vi "T90 konfig.vi"() -> ()   [LabVIEW 2020, in "T90.lvlib"]
uses:
  T90.lvlib
  Visualisierungs Elemente/Auswahlfeld.ctl
  Visualisierungs Elemente/Zahlen-Eingabefeld.ctl
  Zustand Auswahl.ctl
  Visualisierungs Elemente/String - Eingabefeld.ctl
  Visualisierungs Elemente/Pfad-Eingabefeld.ctl
  Seiten/System Einstellungen V2/Konfig Gasflasche.ctl
  Seiten/System Einstellungen V2/Gasflasche Auswahl.ctl
  Seiten/FT-IR/FGV FT-IR Gasliste Aktionen.ctl
  Seiten/System Einstellungen V2/Aktion FGV Gasbottledefinition.ctl
  Aktion FGV T90.ctl
  T90 main.vi
  Seiten/FT-IR/FT-IR.lvlib
  Allgemein/allgemeine Sub-VIs.lvlib
  Sprachverwaltung/Sprachverwaltung.lvlib
  Seiten/System Einstellungen V2/System Einstellungen V2.lvlib
  Linearisierung V2/Gasteiler/Gasteiler.lvlib
panel:
  out "Einheit":string="-22Y3" caption="-21Y8"
  in  "Sollwert:":T1 format="%#_5g"
  in  "Bearbeiter:":T2
  in  "Stabilisierungszeit:":T1 format="%#_5g"
  in  "Gasflasche":T3 items=["----"=10000, "IAG O2"=0, "IAG C2H2"=1, "IAG C2H4"=2, "IAG NH3 200"=3, "IAG NH3 2000"=4, "IAG NH3 3000"=5, "IAG CO 5%"=6, "IAG Propane 2%"=7, "IAG NO 1000"=8, "IAG MG"=9, "IAG SO2"=10, "IAG C3H6"=11, "IAG CO2"=12, "IAG CO"=13, "IAG N2O"=14, "IAG N2O 100"=15, "IAG NO2 1000"=16, "IAG NO2 100"=17, "IAG CH4"=18, "IAG Propane"=19, "IAG NO 5000"=20, "Hansi"=21]
  in  "Konfig Gasflasche":T4 caption="Konfigurierte Gasflasche verwenden"
  in  "max. Responsetime:":T1 format="%#_5g"
  in  "Pfad":T5
  in  "Textname:":T2
  in  "Abschaltzeit:":T1 format="%#_5g"
  in  "Abweichung:":T1 format="%#_5g"
  in  "Abbrechen":bool
  in  "Start":bool
  in  "Modus:":T6=1 items=["Cal Gas", "Entnahmestelle"]
  in  "Gaskomponente:":T7 caption="Komponente:" items=["NO (350,3000) LP 191C", "NO2 (150) LP 191C (1of2)", "NO2 (2000) LP 191C (2of2)", "N2O (300) LP 191C (1of2)", "NH3 (300) LP 191C (1of2)", "NH3 (900,3000) LP 191C (2of2)", "HNCO (400) 191C", "H2O% (30) LP 191C", "Formaldehyde (70,500) LP 191C", "CO2 low% (4) LP 191C (2of2)", "CO2% (20) LP 191C (1of2)", "CO (700) LP 191C (1of3)", "CO% (1) LP 191C (2of3)", "Propylene (1000) LP 191C", "Aromatic HC C7 (500) LP 191C", "Ethylene (1000) LP 191C", "CH4 (250) LP 191C (1of2)", "CH4 (5000) LP 191C (2of2)", "Ethane (1000) LP 191C", "Acetylene (1000) LP 191C", "HNO2 (20) 191C", "MeOH (1000) 191C", "CO% (10) LP 191C (3of3)", "Formic Acid (100) 191C", "SO2 (500) LP 191C", "Acetaldehyde (1000) LP 191C", "COS (100) LP 191C", "1,3 butadiene (100) LP 191C", "Oil as Octane (200) LP 191C", "N2O (1000) LP 191C (2of2)", "Propane (200) LP 191C", "NO2 autorange (2000)", "CO autorange (100000)", "CH4 autorange (5000)", "NH3 autorange (3000)", "NOx autorange (3000)", "HCD (10000)", "NMHCD (10000)", "CO2% autorange (20)", "H2Oppm (300000)", "N2O autorange (1000)", "NMNEHCD (3000)", "Temp. Messzelle", "Druck Messzelle", "sBeam@2500", "Temp. HL zu FT-IR", "Temp. HL Extern SP1", "Austrittstemp. FT-IR", "Temp. Schaltschrank", "Konstant 0", "Konstant 50", "Konstant 100", "AK DUMMY"]
  # "Pfad:"
  # "sec"
  # "%"
  # "T90 Konfig"
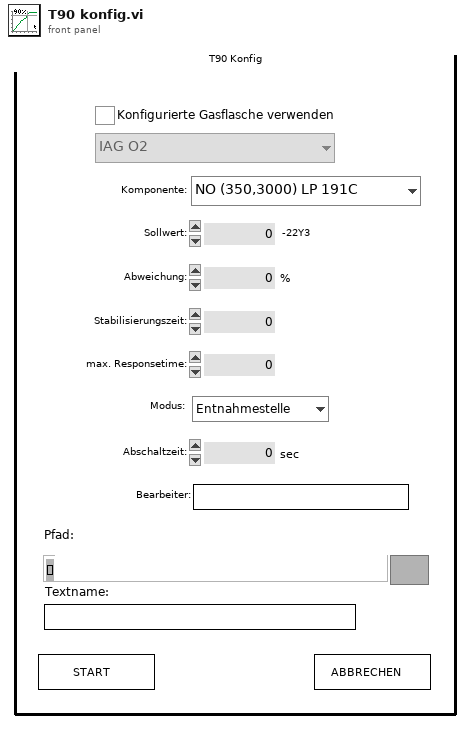
[diagram p1: front panel]
types:
  T1 = typedef "Zahlen-Eingabefeld.ctl" = sgl
  T2 = typedef "String - Eingabefeld.ctl" = string
  T3 = typedef "System Einstellungen V2.lvlib/Gasflasche Auswahl.ctl" = u16
  T4 = typedef "System Einstellungen V2.lvlib/Konfig Gasflasche.ctl" = bool
  T5 = typedef "Pfad-Eingabefeld.ctl" = path
  T6 = typedef "T90.lvlib/Zustand Auswahl.ctl" = u16
  T7 = typedef "Auswahlfeld.ctl" = u16
  T8 = typedef "System Einstellungen V2.lvlib/Aktion FGV Gasbottledefinition.ctl" = enum16{"lesen", "schreiben", "löschen", "laden", "speichern", "exportieren", "importieren"}
  T9 = typedef "FT-IR.lvlib/FGV FT-IR Gasliste Aktionen.ctl" = enum16{"lesen", "Gasliste FT-IR", "Gasliste ausgelesen", "laden", "speichern", "löschen"}
  T10 = typedef "T90.lvlib/Aktion FGV T90.ctl" = enum16{"lesen", "schreiben", "laden", "speichern", "T90 aktiv", "T90 Entnahme aktiv", "Overflow Leak", "Pfad", "Zustand", "max. Responsetime"}
  T11 = typedef "String - Ausgabefeld.ctl" = string
  T12 = typedef "System Einstellungen V2.lvlib/Gasflasche gesamt.ctl" = cluster{"Gasflasche":T13, "Trägergas":T14, "Komponenten":T15[]}
  T13 = typedef "System Einstellungen V2.lvlib/Gasflasche.ctl" = cluster{"Gasname für die Auswahl":string, "Chargennummer":string, "Ablaufdatum":timestamp}
  T14 = typedef "System Einstellungen V2.lvlib/Traegergas.ctl" = string
  T15 = typedef "System Einstellungen V2.lvlib/Gasflaschenkomponente.ctl" = cluster{"Gasauswahl":string, "Konzentration IST":dbl, "Einheit":string, "Genauigkeit":dbl}
  T16 = typedef "T90.lvlib/T90 Gas Konfig.ctl" = cluster{"Gasflasche":T3, "Konfig Gasflasche":T4, "Auswahl":T7, "Sollwert":T1, "Abweichung":T1, "max. Responsetime":T1, "Modus:":T6, "Abschaltzeit":T1, "Stabilisierungszeit":T1, "Bearbeiter":string}
  T17 = cluster{"Komponente:":u16, "Sollwert":dbl, "Accuracy":dbl, "Einheit":string, "Gasflaschen Nr.:":string}
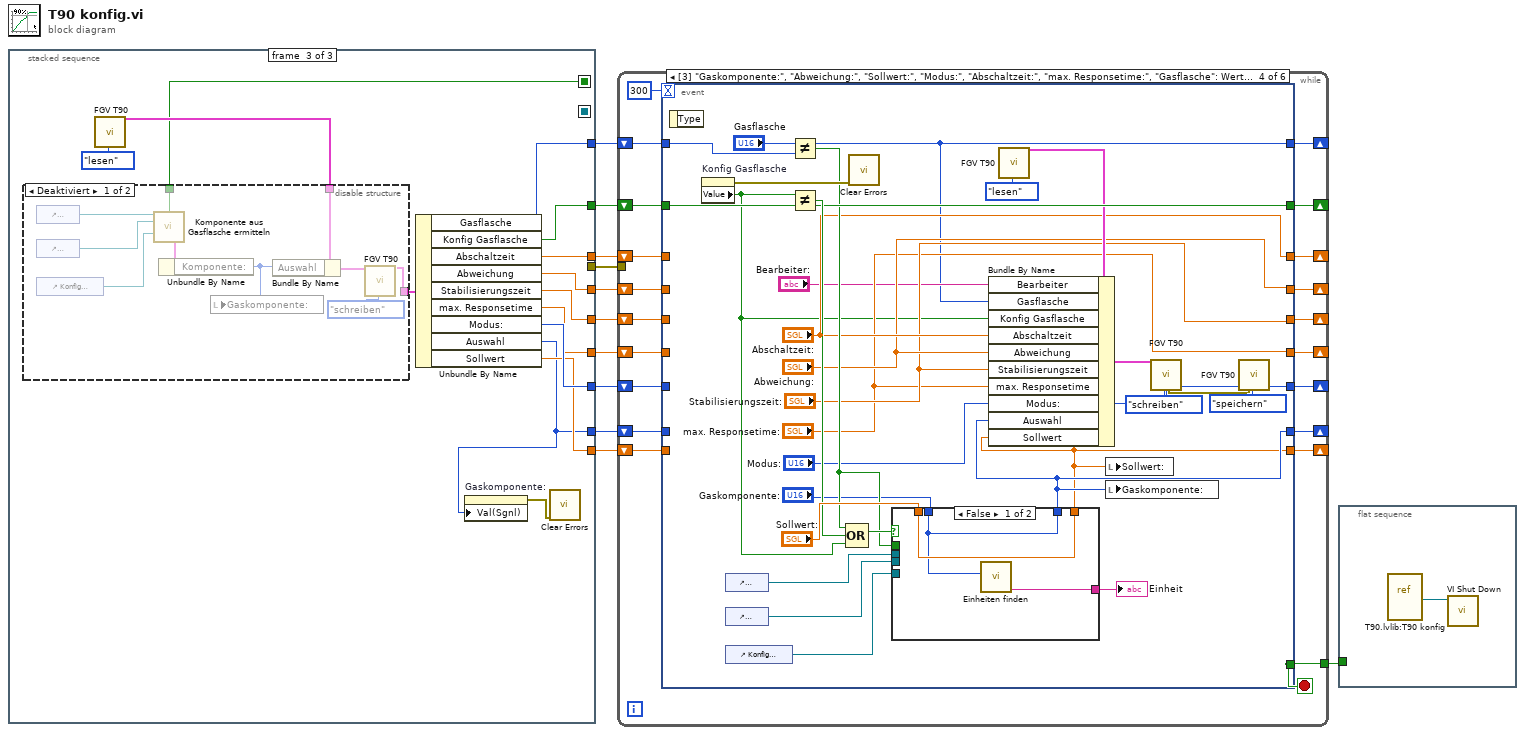
[diagram p0: block diagram]
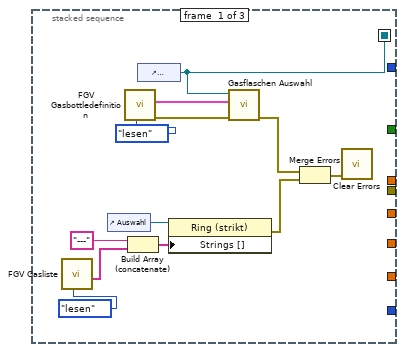
[diagram p2: hidden frame]
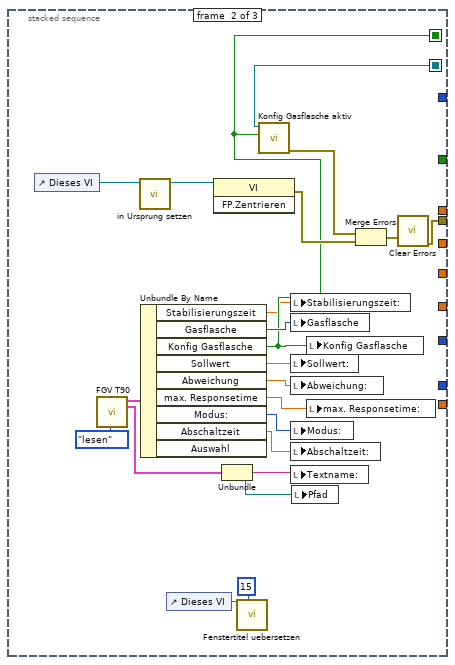
[diagram p3: hidden frame]
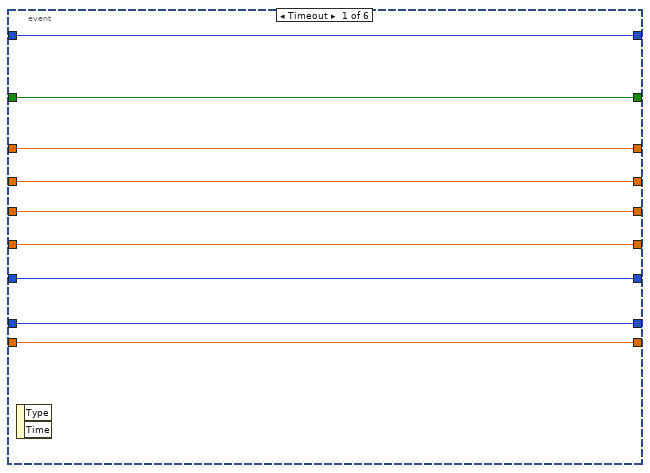
[diagram p5: hidden frame]
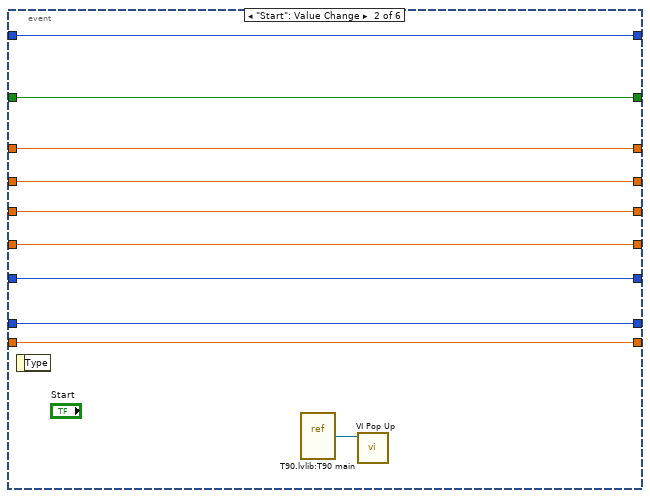
[diagram p6: hidden frame]
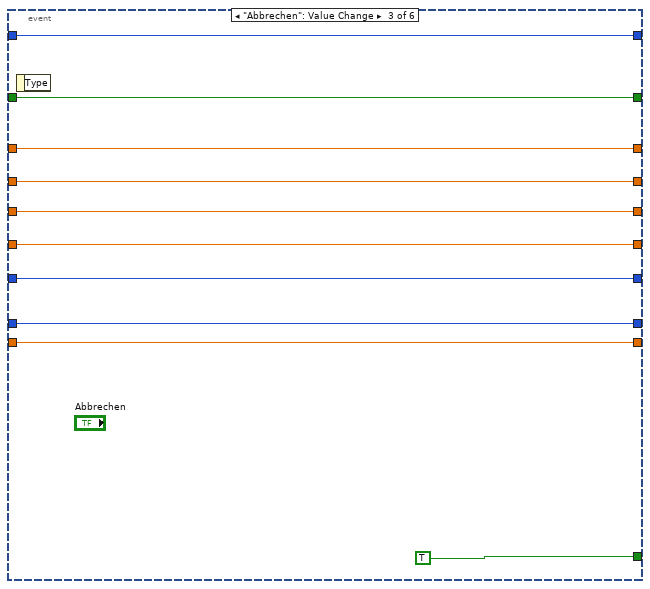
[diagram p7: hidden frame]
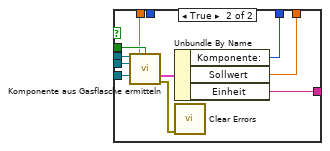
[diagram p8: hidden frame]
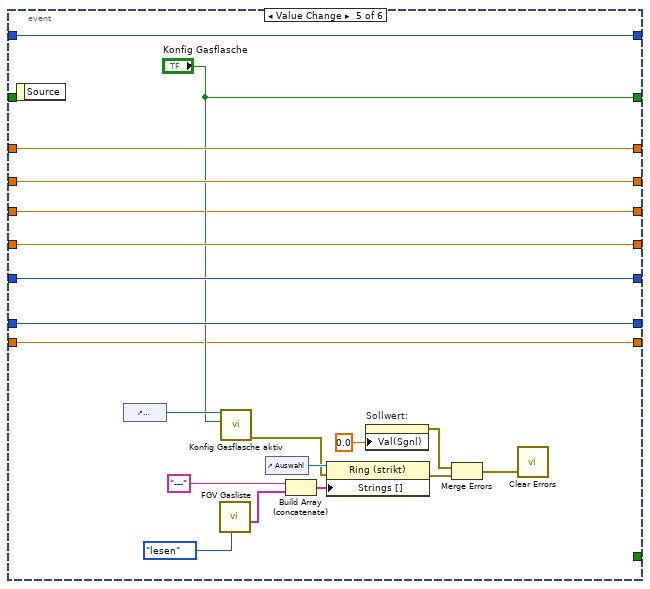
[diagram p9: hidden frame]
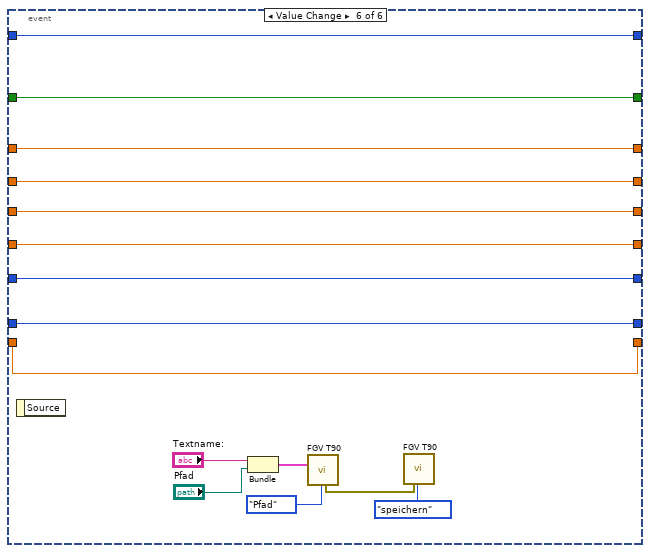
[diagram p10: hidden frame]
diagram:
  n1 = stacked-sequence {
    seq-local: [w15 _ _] -> [_ w27 _]
    seq-local: [_ w26 _] -> [_ _ w57]
    tunnel: [_ w41 _] -> w10
    tunnel: [_ _ w55] -> w9
    tunnel: [_ _ w54] -> w8
    tunnel: [_ _ w53] -> w7
    tunnel: [_ _ w52] -> w6
    tunnel: [_ _ w49] -> w5
    tunnel: [_ _ w51] -> w4
    tunnel: [_ _ w46] -> w3
    tunnel: [_ _ w50] -> w2
    tunnel: [_ _ w48] -> w1
    frame #0 {
      n2 = call "FGV Gasliste.vi"("Aktionen"=FGV_FT-IR_Gasliste_Aktionen."lesen") -> ("Aktuelle Gasliste gesamt"=w20:T11[])  [unwired: 8 in, 2 out]
      n3 = control-ref of="Auswahl"() -> (w22:refnum<vi>)
      n4 = call "FGV Gasbottledefinition.vi"("Aktion"=Aktion_FGV_Gasbottledefinition."lesen") -> ("error out"=w18:errorcluster, "Gasflaschen Liste gesamt"=w17:T12[])  [unwired: 8 in, 1 out]
      n5 = Build Array (concatenate)("---", w20) -> (w23:T11[])
      n6 = control-ref of="Gasflasche"() -> (w15:refnum<vi>)
      n7 = property class="Ring (strikt)"(reference=w22, "Strings []"=w23) -> (error out=w14:errorcluster)  [unwired: 1 in, 1 out]
      n8 = call "Gasflaschen Auswahl.vi"("error in (no error)"=w18, "Gasflaschen Liste gesamt"=w17, "Ring (Eingang)"=w15) -> ("error out"=w13:errorcluster)  [unwired: 8 in]
      n9 = Merge Errors(w13, w14) -> (w12:errorcluster)
      n10 = call <vilib>:"Clear Errors.vi"("error in (no error)"=w12) -> ()  [unwired: 5 in, 2 out]
    }
    frame #1 {
      n11 = control-ref of="Dieses VI"() -> (w44:refnum<vi>)
      n12 = call "FGV T90.vi"("Aktion"=Aktion_FGV_T90."lesen") -> ("Gas Konfig"=w35:T16, "Protokolldaten"=w38:cluster{"File Name":T2, "Pfad":T5})  [unwired: 20 in, 5 out]
      n13 = call "in Ursprung setzen.vi"("VI Referenz"=w44) -> ("Referenz (Ausgang)"=w24:refnum<vi>)  [unwired: 10 in]
      n14 = Unbundle By Name(w35) -> ("Stabilisierungszeit"=w25:T1, "Gasflasche"=w34:T3, "Konfig Gasflasche"=w26:T4, "Sollwert"=w33:T1, "Abweichung"=w32:T1, "max. Responsetime"=w31:T1, "Modus:"=w30:T6, "Abschaltzeit"=w29:T1)  [unwired: 1 out]
      n15 = control-ref of="Dieses VI"() -> (w39:refnum<vi>)
      n16 = invoke class="VI" method="FP.Zentrieren"(reference=w24) -> (error out=w43:errorcluster)  [unwired: 2 in, 2 out]
      n17 = Unbundle(w38) -> ("File Name"=w37:T2, "Pfad"=w36:T5)
      n18 = call "Fenstertitel uebersetzen.vi"("Index (Seite)"=15, "Dieses VI"=w39) -> ()  [unwired: 6 in, 4 out]
      n19 = call "Konfig Gasflasche aktiv.vi"("Konfig Gasflasche"=w26, "Referenz Gasflasche"=w27) -> ("error out"=w28:errorcluster)  [unwired: 9 in]
      n20 = local write "Stabilisierungszeit:"(w25) -> ()
      n21 = local write "Gasflasche"(w34) -> ()
      n22 = local write "Sollwert:"(w33) -> ()
      n23 = local write "Abweichung:"(w32) -> ()
      n24 = local write "Modus:"(w30) -> ()
      n25 = local write "Abschaltzeit:"(w29) -> ()
      n26 = local write "Textname:"(w37) -> ()
      n27 = local write "Pfad"(w36) -> ()
      n28 = local write "Konfig Gasflasche"(w26) -> ()
      n29 = local write "max. Responsetime:"(w31) -> ()
      n30 = Merge Errors(w28, w43) -> (w42:errorcluster)
      n31 = call <vilib>:"Clear Errors.vi"("error in (no error)"=w42) -> ("error out"=w41:errorcluster)  [unwired: 5 in, 1 out]
    }
    frame #2 {
      n32 = call "FGV T90.vi"("Aktion"=Aktion_FGV_T90."lesen") -> ("Gas Konfig"=w58:T16)  [unwired: 20 in, 6 out]
      n33 = disable-structure shown="Deaktiviert" {
        disable-tunnel: w58 -> [w65 w70]
        disable-tunnel: w57 -> [w61 _]
        disable-tunnel: [w60 w70] -> w56
        frame Disabled {
          n34 = control-ref of="Gasflasche"() -> (w69:refnum<vi>)
          n35 = control-ref of="Gaskomponente:"() -> (w68:refnum<vi>)
          n36 = control-ref of="Konfig Gasflasche"() -> (w67:refnum<vi>)
          n37 = call "Komponente aus Gasflasche ermitteln.vi"("Referenz Gasflasche"=w69, "Wertänderung Gasflasche"=w61, "Referenz Komponente"=w68, "Referenz Konfig Gasflasche"=w67) -> ("Ausgangs-Cluster"=w66:T17)  [unwired: 8 in, 3 out]
          n38 = Unbundle By Name(w66) -> ("Komponente:"=w62:u16)
          n39 = local write "Gaskomponente:"(w62) -> ()
          n40 = Bundle By Name(cluster=w65, "Auswahl"=w62) -> (w63:T16)
          n41 = call "FGV T90.vi"("Gas Konfig"=w63, "Aktion"=Aktion_FGV_T90."schreiben") -> ("Gas Konfig"=w60:T16)  [unwired: 19 in, 6 out]
        }
        frame Enabled {
        }
      }
      n42 = Unbundle By Name(w56) -> ("Gasflasche"=w55:T3, "Konfig Gasflasche"=w54:T4, "Abschaltzeit"=w53:T1, "Abweichung"=w52:T1, "Stabilisierungszeit"=w48:T1, "max. Responsetime"=w49:T1, "Modus:"=w51:T6, "Auswahl"=w46:T7, "Sollwert"=w50:T1)
      n43 = property on="Gaskomponente:" class="Ring (strikt)"("Val(Sgnl)"=w46) -> (error out=w47:errorcluster)  [unwired: 2 in, 1 out]
      n44 = call <vilib>:"Clear Errors.vi"("error in (no error)"=w47) -> ()  [unwired: 5 in, 2 out]
    }
  }
  n45 = while {
    tunnel: [w89] -> w11
    shift-right: [w88] -> _
    shift-left: w2 -> [w87]
    shift-right: [w86] -> _
    shift-left: w6 -> [w83]
    shift-right: [w85] -> _
    shift-left: w4 -> [w82]
    shift-right: [w84] -> _
    shift-left: w3 -> [w81]
    shift-right: [w80] -> _
    shift-left: w7 -> [w79]
    tunnel: w10 -> [_]
    shift-right: [w78] -> _
    shift-left: w5 -> [w77]
    shift-right: [w76] -> _
    shift-left: w9 -> [w73]
    shift-right: [w75] -> _
    shift-left: w8 -> [w74]
    shift-right: [w71] -> _
    shift-left: w1 -> [w72]
    stop <- w89 stop-if-true
    n46 = event shown="[3] \"Gaskomponente:\", \"Abweichung:\", \"Sollwert:\", \"Modus:\", \"Abschaltzeit:\", \"max. Responsetime:\", \"Gasflasche\": Wertänderung" {
      selector: _ -> [_ _ _ _ _ _]
      dyn-events: _ -> [_ _ _ _ _ _]
      timeout: 300 -> [_ _ _ _ _ _]
      tunnel: [_ _ TRUE _ _ _] -> w89
      tunnel: [w98 w107 w115 w131 w166 w185] -> w88
      tunnel: w87 -> [w98 w107 w115 _ w166 w185]
      tunnel: [w97 w106 w116 "Abweichung:" w177 w186] -> w86
      tunnel: [w96 w105 w118 "Modus:" w175 w188] -> w85
      tunnel: [w95 w104 w117 w132 w174 w189] -> w84
      tunnel: w83 -> [w97 w106 w116 _ w177 w186]
      tunnel: w82 -> [w96 w105 w118 _ w175 w188]
      tunnel: w81 -> [w95 w104 w117 _ w174 w189]
      tunnel: [w99 w108 w114 "Abschaltzeit:" w178 w184] -> w80
      tunnel: w79 -> [w99 w108 w114 _ w178 w184]
      tunnel: [w94 w103 w113 "max. Responsetime:" w176 w187] -> w78
      tunnel: w77 -> [w94 w103 w113 _ w176 w187]
      tunnel: [w93 w102 w111 "Gasflasche" w179 w182] -> w76
      tunnel: [w92 w101 w112 w139 "Konfig Gasflasche" w183] -> w75
      tunnel: w74 -> [w92 w101 w112 w139 _ w183]
      tunnel: w73 -> [w93 w102 w111 w141 w179 w182]
      tunnel: w72 -> [w91 w100 w110 _ w161 w181]
      tunnel: [w91 w100 w110 "Stabilisierungszeit:" w161 w181] -> w71
      event Timeout {
        n47 = event-data() -> ()  [unwired: 1 in, 2 out]
      }
      event "Start": Value Change {
        n48 = event-data() -> ()  [unwired: 1 in, 1 out]
        n49 = vi-ref "T90.lvlib:T90 main.vi"() -> (w109:refnum<vi>)
        n50 = call "VI Pop Up.vi"("VI Referenz"=w109) -> ()  [unwired: 10 in, 1 out]
      }
      event "Abbrechen": Value Change {
        n51 = event-data() -> ()  [unwired: 1 in, 1 out]
      }
      event Value Change {
        n52 = event-data() -> ()  [unwired: 1 in, 1 out]
        n53 = property on="Konfig Gasflasche" class="Bool. (strikt)"() -> (error out=w140:errorcluster, "Value"=w121:T4)  [unwired: 2 in, 1 out]
        n54 = control-ref of="Gasflasche"() -> (w146:refnum<vi>)
        n55 = control-ref of="Gaskomponente:"() -> (w144:refnum<vi>)
        n56 = control-ref of="Konfig Gasflasche"() -> (w145:refnum<vi>)
        n57 = Not Equal?(x="Gasflasche", y=w141) -> (x != y?=w137:bool)
        n58 = Not Equal?(x=w121, y=w139) -> (x != y?=w142:T4)
        n59 = Compound Arithmetic op=OR ("Mehrfacharithmetik")(w137, w142, w121) -> (w138:T4)
        n60 = call <vilib>:"Clear Errors.vi"("error in (no error)"=w140) -> ()  [unwired: 5 in, 2 out]
        n61 = case shown="False" w138 {
          tunnel: w146 -> [_ w159]
          tunnel: w145 -> [_ w158]
          tunnel: w144 -> [_ w157]
          tunnel: [w149 w156] -> w132
          tunnel: [w150 w153] -> w131
          tunnel: "Gaskomponente:" -> [w149 _]
          tunnel: "Sollwert:" -> [w150 w151]
          tunnel: w137 -> [_ w154]
          tunnel: [w148 w152] -> w120
          frame False {
            n62 = call "Einheiten finden.vi"("Komponente"=w149) -> ("Einheit in String"=w148:string)  [unwired: 6 in, 4 out]
          }
          frame True {
            n63 = call "Komponente aus Gasflasche ermitteln.vi"("Referenz Gasflasche"=w159, "Konzentration IST"=w151, "Wertänderung Gasflasche"=w154, "Referenz Komponente"=w157, "Referenz Konfig Gasflasche"=w158) -> ("Ausgangs-Cluster"=w160:T17, "error out"=w155:errorcluster)  [unwired: 7 in, 2 out]
            n64 = Unbundle By Name(w160) -> ("Komponente:"=w156:u16, "Sollwert"=w153:dbl, "Einheit"=w152:string)
            n65 = call <vilib>:"Clear Errors.vi"("error in (no error)"=w155) -> ()  [unwired: 5 in, 2 out]
          }
        }
        "Einheit" <- w120
        n66 = call "FGV T90.vi"("Aktion"=Aktion_FGV_T90."lesen") -> ("Gas Konfig"=w135:T16)  [unwired: 20 in, 6 out]
        n67 = Bundle By Name(cluster=w135, "Bearbeiter"="Bearbeiter:", "Gasflasche"="Gasflasche", "Konfig Gasflasche"=w121, "Abschaltzeit"="Abschaltzeit:", "Abweichung"="Abweichung:", "Stabilisierungszeit"="Stabilisierungszeit:", "max. Responsetime"="max. Responsetime:", "Modus:"="Modus:", "Auswahl"=w132, "Sollwert"=w131) -> (w130:T16)
        n68 = local write "Sollwert:"(w131) -> ()
        n69 = local write "Gaskomponente:"(w132) -> ()
        n70 = call "FGV T90.vi"("Gas Konfig"=w130, "Aktion"=Aktion_FGV_T90."schreiben") -> ("error out"=w127:errorcluster)  [unwired: 19 in, 6 out]
        n71 = call "FGV T90.vi"("error in (no error)"=w127, "Aktion"=Aktion_FGV_T90."speichern") -> ()  [unwired: 19 in, 7 out]
      }
      event Value Change {
        n72 = event-data() -> ()  [unwired: 1 in, 1 out]
        n73 = control-ref of="Gasflasche"() -> (w180:refnum<vi>)
        n74 = call "FGV Gasliste.vi"("Aktionen"=FGV_FT-IR_Gasliste_Aktionen."lesen") -> ("Aktuelle Gasliste gesamt"=w172:T11[])  [unwired: 8 in, 2 out]
        n75 = call "Konfig Gasflasche aktiv.vi"("Konfig Gasflasche"="Konfig Gasflasche", "Referenz Gasflasche"=w180) -> ("error out"=w167:errorcluster)  [unwired: 9 in]
        n76 = control-ref of="Auswahl"() -> (w168:refnum<vi>)
        n77 = Build Array (concatenate)("---", w172) -> (w171:T11[])
        n78 = property class="Ring (strikt)"(reference=w168, error in=w167, "Strings []"=w171) -> (error out=w163:errorcluster)  [unwired: 1 out]
        n79 = property on="Sollwert:" class="DigWert (strikt)"("Val(Sgnl)"=T1 0.0 ("Wert (signalisierend)")) -> (error out=w164:errorcluster)  [unwired: 2 in, 1 out]
        n80 = Merge Errors(w164, w163) -> (w162:errorcluster)
        n81 = call <vilib>:"Clear Errors.vi"("error in (no error)"=w162) -> ()  [unwired: 5 in, 2 out]
      }
      event Value Change {
        n82 = event-data() -> ()  [unwired: 1 in, 1 out]
        n83 = Bundle("Textname:"="Textname:", "Pfad"="Pfad") -> (w195:cluster{"Textname:":T2, "Pfad":T5})  [unwired: 1 in]
        n84 = call "FGV T90.vi"("Protokolldaten"=w195, "Aktion"=Aktion_FGV_T90."Pfad") -> ("error out"=w194:errorcluster)  [unwired: 19 in, 6 out]
        n85 = call "FGV T90.vi"("error in (no error)"=w194, "Aktion"=Aktion_FGV_T90."speichern") -> ()  [unwired: 19 in, 7 out]
      }
    }
  }
  n86 = flat-sequence {
    tunnel: w11 -> [_]
    frame #0 {
      n87 = vi-ref "T90.lvlib:T90 konfig.vi"() -> (w196:refnum<vi>)
      n88 = call "VI Shut Down.vi"("VI Referenz"=w196) -> ()  [unwired: 11 in]
    }
  }
